vi "Channel Manager.vi"(7 "action":T2, 8 "error in":errorcluster, 10 "channel number":u8, 11 "board handle":u8) -> (0 "error out":errorcluster, 1 "channel info":cluster{"count":u32, "status":T1}, 2 "channel number out":u8, 3 "board handle out":u8)   [LabVIEW 2024, in "AIM ARINC 429 Hardware API.lvlib"]
uses:
  AIM ARINC 429 Hardware API.lvlib
  Channel Action.ctl
  Channel Status.ctl
  <vilib>/Utility/miscctls.llb/LVMapReplaceAction.ctl
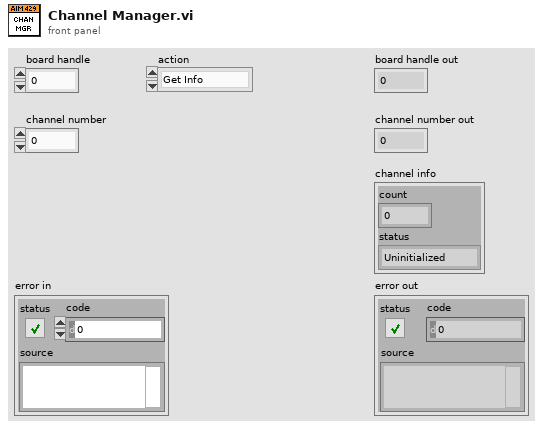
[diagram p1: front panel]
types:
  T1 = typedef "AIM ARINC 429 Hardware API.lvlib/Channel Status.ctl" = enum16{"Uninitialized", "Idle", "Active"}
  T2 = typedef "AIM ARINC 429 Hardware API.lvlib/Channel Action.ctl" = enum16{"Get Info", "Initialize", "Start", "Clear"}
  T3 = map{cluster{"board handle":u8, "channel number":u8}, cluster{"count":u32, "status":T1}}
  T4 = typedef "LVMapReplaceAction.ctl" = enum32{"Modify Entry only if found", "Add or Modify Entry", "Delete Entry"}
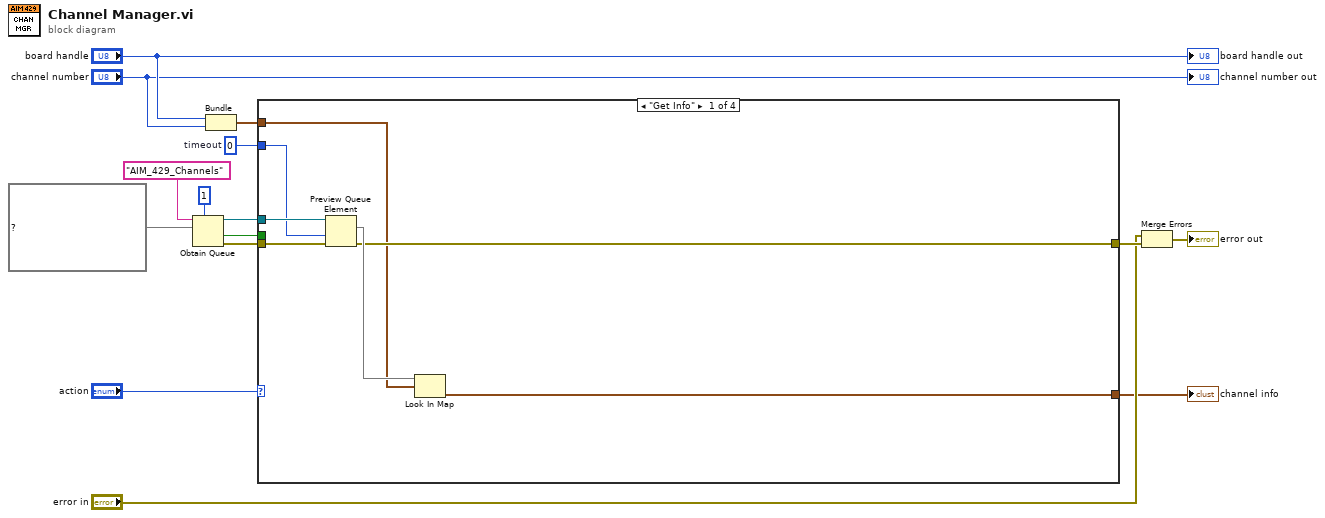
[diagram p0: block diagram]
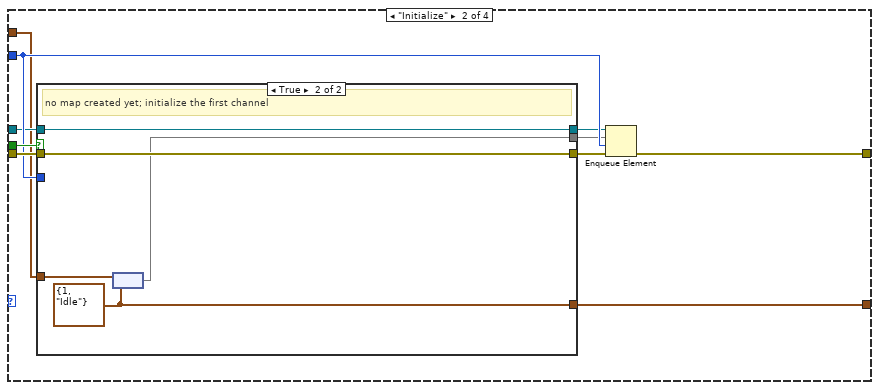
[diagram p2: hidden frame]
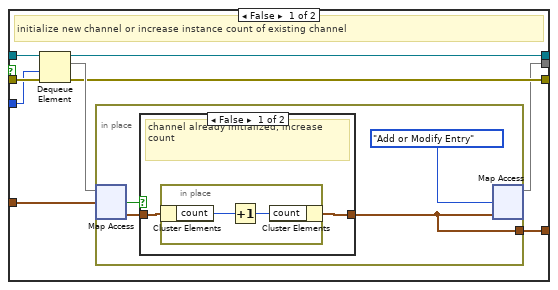
[diagram p3: hidden frame]
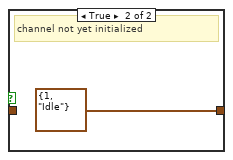
[diagram p4: hidden frame]
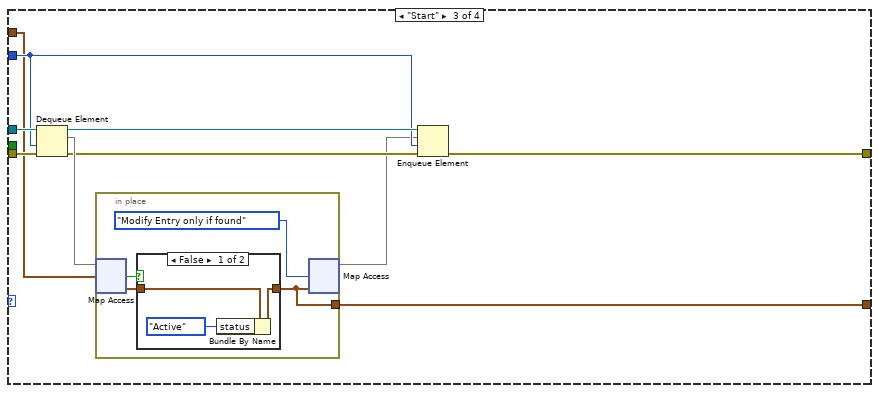
[diagram p5: hidden frame]
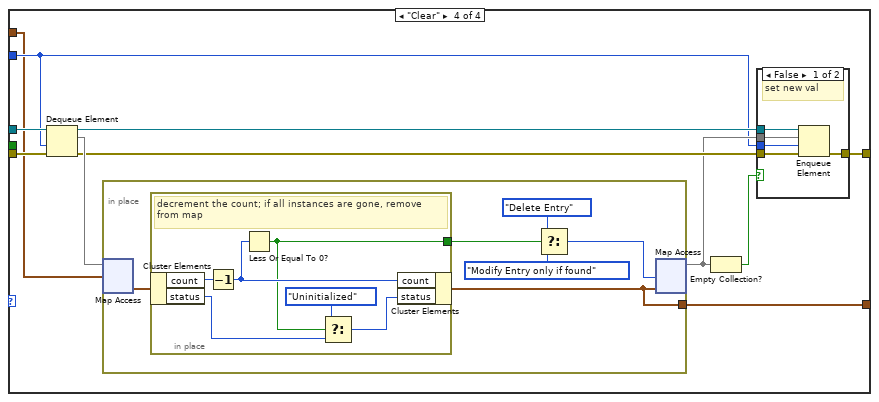
[diagram p7: hidden frame]
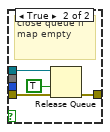
[diagram p8: hidden frame]
diagram:
  w6 = 0  # timeout
  n1 = Obtain Queue(max queue size (-1, unlimited)=1, name (unnamed)="AIM_429_Channels", element data type=T3 {} ("channel counter")) -> (queue out=w9:refnum<queue>, created new?=w8:bool, error out=w7:errorcluster)  [unwired: 2 in]
  n2 = Bundle("board handle"="board handle", "channel number"="channel number") -> (w1:cluster{"board handle":u8, "channel number":u8})  [unwired: 1 in]
  n3 = case shown="\"Get Info\"" "action" {
    tunnel: w9 -> [w21 w28 w63 w82]
    tunnel: w8 -> [_ w31 _ _]
    tunnel: w7 -> [w22 w30 w64 w83]
    tunnel: w6 -> [w20 w29 w59 w75]
    tunnel: [w18 w26 w58 w78] -> w5
    tunnel: [w17 w24 w56 w74] -> w2
    tunnel: w1 -> [w16 w23 w55 w73]
    frame "Get Info" {
      n4 = Preview Queue Element(queue=w21, timeout in ms (-1)=w20, error in (no error)=w22) -> (element=w19:T3, error out=w18:errorcluster)  [unwired: 2 out]
      n5 = Look In Map(map=w19, key=w16) -> (value=w17:cluster{"count":u32, "status":T1})  [unwired: 1 in, 1 out]
    }
    frame "Initialize" {
      n6 = case shown="True" w31 {
        tunnel: w30 -> [w40 w53]
        tunnel: w29 -> [w39 _]
        tunnel: w28 -> [w38 w52]
        tunnel: w23 -> [w36 w54]
        tunnel: [w35 w53] -> _
        tunnel: [w33 w51] -> w27
        tunnel: [w34 w52] -> w25
        tunnel: [w32 w50] -> w24
        frame False {
          # "initialize new channel or increase instance count of existing channel"
          n7 = Dequeue Element(queue=w38, timeout in ms (-1)=w39, error in (no error)=w40) -> (queue out=w34:refnum<queue>, element=w37:T3, error out=w35:errorcluster)  [unwired: 1 out]
          n8 = in-place {
            in-place-border: [w41] -> w32
            n9 = in-place-map #1(w37, w36) -> (w43:cluster{"count":u32, "status":T1}, w44:bool)  [unwired: 1 in]
            n10 = case shown="False" w44 {
              tunnel: w43 -> [w46 _]
              tunnel: [w45 cluster{"count":u32, "status":T1} {"count"=1, "status"=enum."Idle"}] -> w41
              frame False {
                # "channel already initialized; increase count"
                n11 = in-place {
                  n12 = in-place-cluster #2(w46) -> ("count"=w48:u32)
                  n13 = Increment(x=w48) -> (x+1=w47:u32)
                  n14 = in-place-cluster #2("count"=w47) -> (w45:cluster{"count":u32, "status":T1})
                }
              }
              frame True {
                # "channel not yet initialized"
              }
            }
            n15 = in-place-map #1(w41, LVMapReplaceAction."Add or Modify Entry" ("action")) -> (w33:T3)  [unwired: 2 out]
          }
        }
        frame True {
          w50 = cluster{"count":u32, "status":T1} {"count"=1, "status"=enum."Idle"}
          # "no map created yet; initialize the first channel"
          n16 = node(w54, w50) -> (w51:T3)
        }
      }
      n17 = Enqueue Element(queue=w25, element=w27, timeout in ms (-1)=w29, error in (no error)=w30) -> (error out=w26:errorcluster)  [unwired: 2 out]
    }
    frame "Start" {
      n18 = Dequeue Element(queue=w63, timeout in ms (-1)=w59, error in (no error)=w64) -> (queue out=w60:refnum<queue>, element=w62:T3, error out=w61:errorcluster)  [unwired: 1 out]
      n19 = in-place {
        in-place-border: [w65] -> w56
        n20 = in-place-map #3(w62, w55) -> (w68:cluster{"count":u32, "status":T1}, w66:bool)  [unwired: 1 in]
        n21 = case shown="False" w66 {
          tunnel: w68 -> [w71 w72]
          tunnel: [w69 w72] -> w65
          frame False {
            n22 = Bundle By Name(cluster=w71, "status"=Channel_Status."Active") -> (w69:cluster{"count":u32, "status":T1})
          }
          frame True {
          }
        }
        n23 = in-place-map #3(w65, LVMapReplaceAction."Modify Entry only if found" ("action")) -> (w57:T3)  [unwired: 2 out]
      }
      n24 = Enqueue Element(queue=w60, element=w57, timeout in ms (-1)=w59, error in (no error)=w61) -> (error out=w58:errorcluster)  [unwired: 2 out]
    }
    frame "Clear" {
      n25 = Dequeue Element(queue=w82, timeout in ms (-1)=w75, error in (no error)=w83) -> (queue out=w79:refnum<queue>, element=w81:T3, error out=w80:errorcluster)  [unwired: 1 out]
      n26 = in-place {
        in-place-border: [w93] -> w74
        n27 = in-place-map #4(w81, w73) -> (w98:cluster{"count":u32, "status":T1})  [unwired: 1 in, 1 out]
        n28 = in-place {
          in-place-border: [w102] -> w94
          # "decrement the count; if all instances are gone, remove from map"
          n29 = in-place-cluster #5(w98) -> ("count"=w104:u32, "status"=w101:T1)
          n30 = Decrement(x=w104) -> (x-1=w103:u32)
          n31 = Less Or Equal To 0?(x=w103) -> (x <= 0?=w102:bool)
          n32 = Select(t=Channel_Status."Uninitialized", s=w102, f=w101) -> (s? t:f=w100:T1)
          n33 = in-place-cluster #5("count"=w103, "status"=w100) -> (w93:cluster{"count":u32, "status":T1})
        }
        n34 = Select(t=LVMapReplaceAction."Delete Entry" ("action"), s=w94, f=LVMapReplaceAction."Modify Entry only if found" ("action")) -> (s? t:f=w95:T4)
        n35 = in-place-map #4(w93, w95) -> (w76:T3)  [unwired: 2 out]
      }
      n36 = Empty Collection?(1:w76) -> (0:w77:bool)
      n37 = case shown="False" w77 {
        tunnel: w80 -> [w88 w92]
        tunnel: w79 -> [w87 w91]
        tunnel: [w86 w90] -> w78
        tunnel: w76 -> [w85 _]
        tunnel: w75 -> [w84 _]
        frame False {
          # "set new val"
          n38 = Enqueue Element(queue=w87, element=w85, timeout in ms (-1)=w84, error in (no error)=w88) -> (error out=w86:errorcluster)  [unwired: 2 out]
        }
        frame True {
          # "close queue if map empty"
          n39 = Release Queue(queue=w91, force destroy? (F)=TRUE, error in (no error)=w92) -> (error out=w90:errorcluster)  [unwired: 2 out]
        }
      }
    }
  }
  "channel info" <- w2
  n40 = Merge Errors("error in", w5) -> (→"error out":errorcluster)
  "board handle out" <- "board handle"
  "channel number out" <- "channel number"
